vi "main.vi"() -> ()   [LabVIEW 2023, in "Vending_machine.lvlib"]
doc: "A vending machine"
uses:
  Vending_machine.lvlib
  Queue Opertaions.ctl
  Controls/Machine_data.ctl
  Controls/Cash.ctl
  Controls/Panel_states.ctl
  Controls/Read_Write.ctl
  <vilib>/Utility/error.llb/DialogType.ctl
  <vilib>/Utility/error.llb/Error Cluster From Error Code.vi
  <vilib>/ErrorRing/Error Ring.xnode
panel:
  in  "Gen_error":bool
  out "error out":errorcluster
  in  "error in (no error)":errorcluster
  in  "Reset Machine":bool
  out "Total cash":i32
  out "Total No. of cans":i32
  in  "Open Door":bool
  out "LED":bool
  in  "Cancel":bool
  in  "Sprite":bool
  in  "Fanta":bool
  in  "Coke":bool
  out "msg_box":string
  in  "5":bool
  in  "10":bool
  in  "20":bool
  in  "50":bool
  in  "100":bool
  # "Cash Selection"
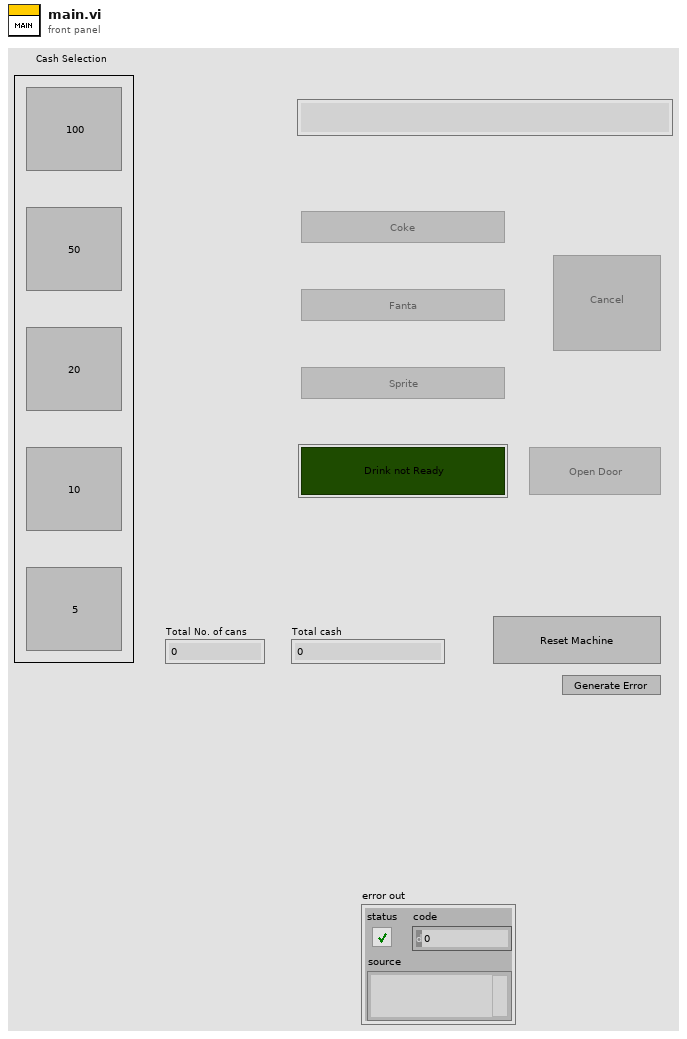
[diagram p1: front panel]
types:
  T1 = typedef "Vending_machine.lvlib/Queue Opertaions.ctl" = enum16{"Create", "Enqueue", "Enqueue N", "Flush", "Dequeue", "Destroy"}
  T2 = typedef "Vending_machine.lvlib/Machine_data.ctl" = cluster{"Cash":T3, "Panel_State":T4, "User_Cash":T3, "Drink":string, "Can_Count":i32, "Message_box":string, "LED":bool, "Last_Activity":timestamp, "Cash remaining":T3, "Drink_price":i32, "No_Activity_Limit(s)":dbl}
  T3 = typedef "Vending_machine.lvlib/Cash.ctl" = cluster{"100":i32, "50":i32, "20":i32, "10":i32, "5":i32}
  T4 = typedef "Vending_machine.lvlib/Panel_states.ctl" = cluster{"100":enum8{"Enabled", "Disabled", "Disabled and Grayed Out"}, "50":enum8{"Enabled", "Disabled", "Disabled and Grayed Out"}, "20":enum8{"Enabled", "Disabled", "Disabled and Grayed Out"}, "10":enum8{"Enabled", "Disabled", "Disabled and Grayed Out"}, "5":enum8{"Enabled", "Disabled", "Disabled and Grayed Out"}, "Cancel":enum8{"Enabled", "Disabled", "Disabled and Grayed Out"}, "Coke":enum8{"Enabled", "Disabled", "Disabled and Grayed Out"}, "Sprite":enum8{"Enabled", "Disabled", "Disabled and Grayed Out"}, "Fanta":enum8{"Enabled", "Disabled", "Disabled and Grayed Out"}, "Open_Door":enum8{"Enabled", "Disabled", "Disabled and Grayed Out"}}
  T5 = enum8{"Enabled", "Disabled", "Disabled and Grayed Out"}
  T6 = typedef "Vending_machine.lvlib/Read_Write.ctl" = enum16{"Read", "Write"}
  T7 = typedef "DialogType.ctl" = u16
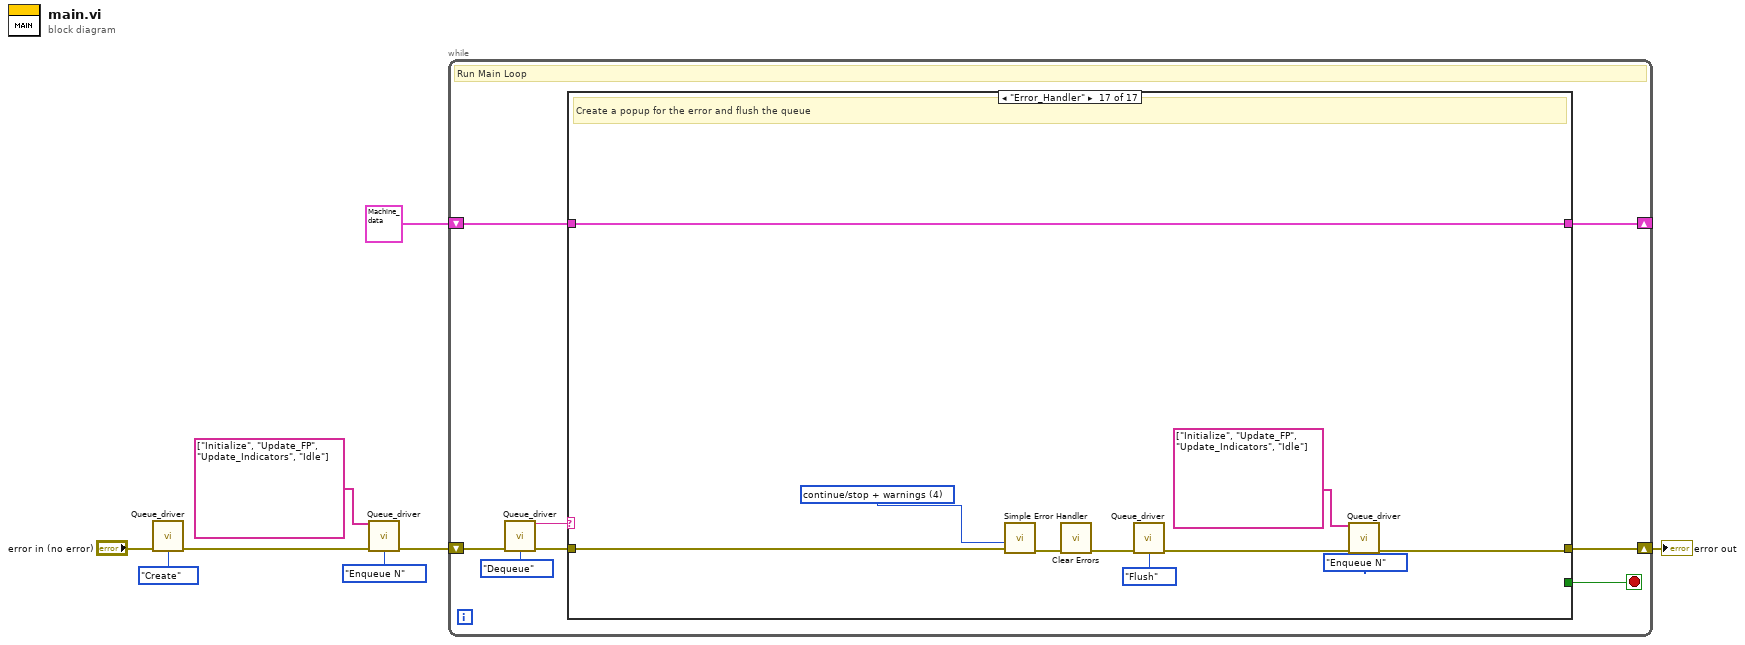
[diagram p0: block diagram]
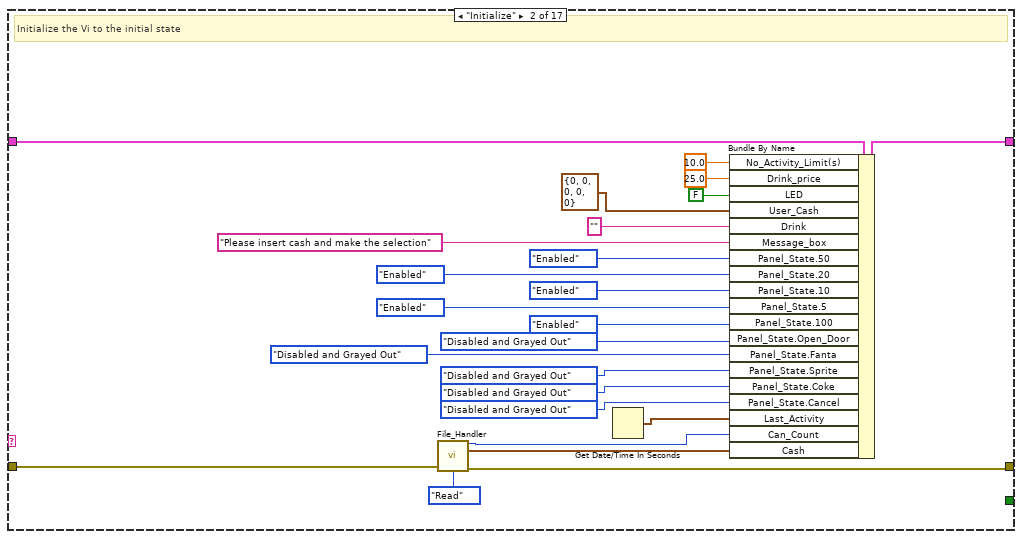
[diagram p3: hidden frame]
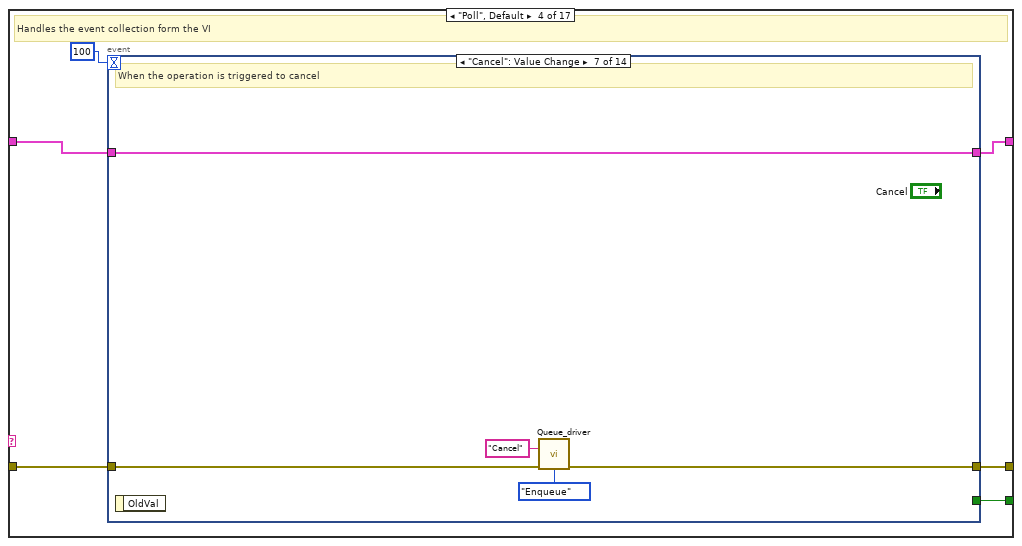
[diagram p5: hidden frame]
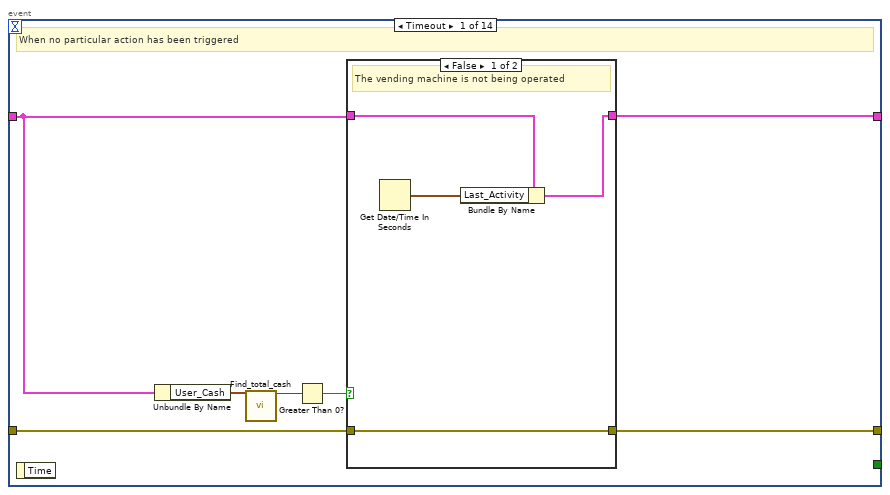
[diagram p6: hidden frame]
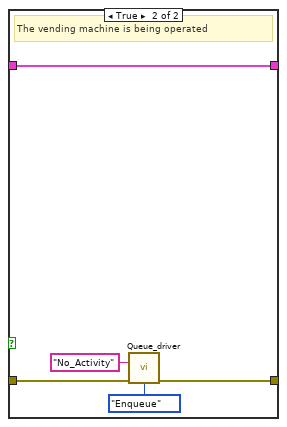
[diagram p7: hidden frame]
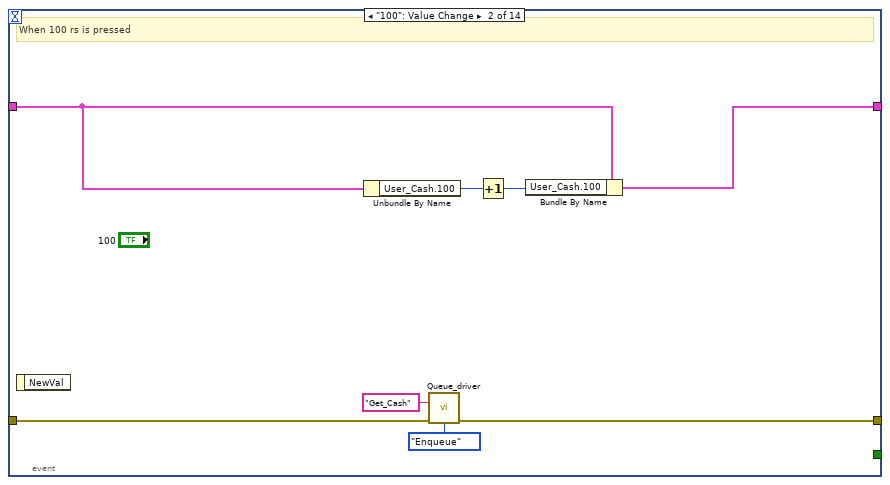
[diagram p8: hidden frame]
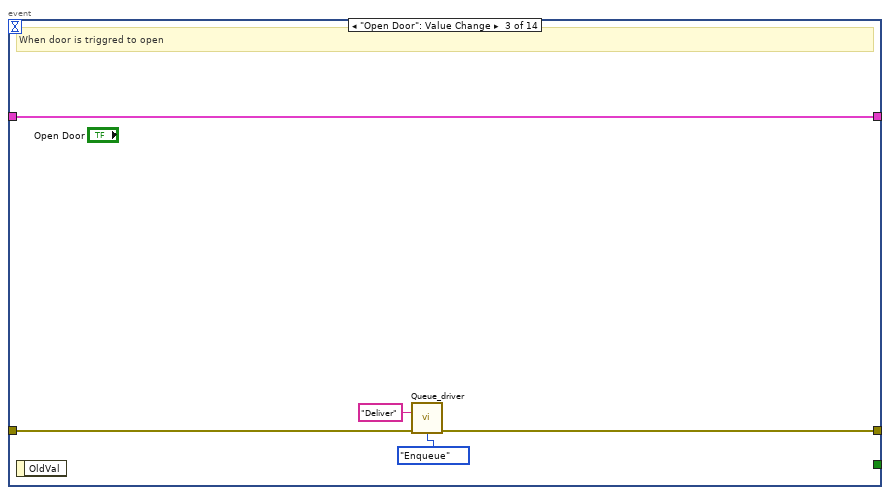
[diagram p9: hidden frame]
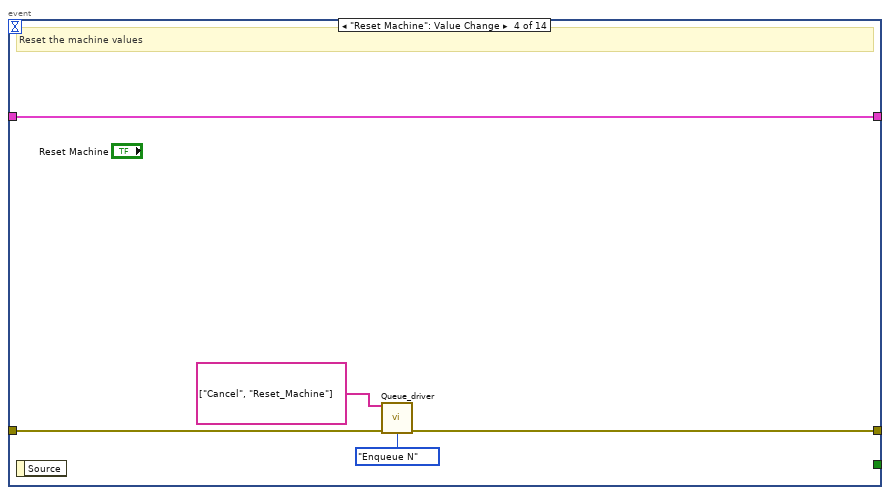
[diagram p10: hidden frame]
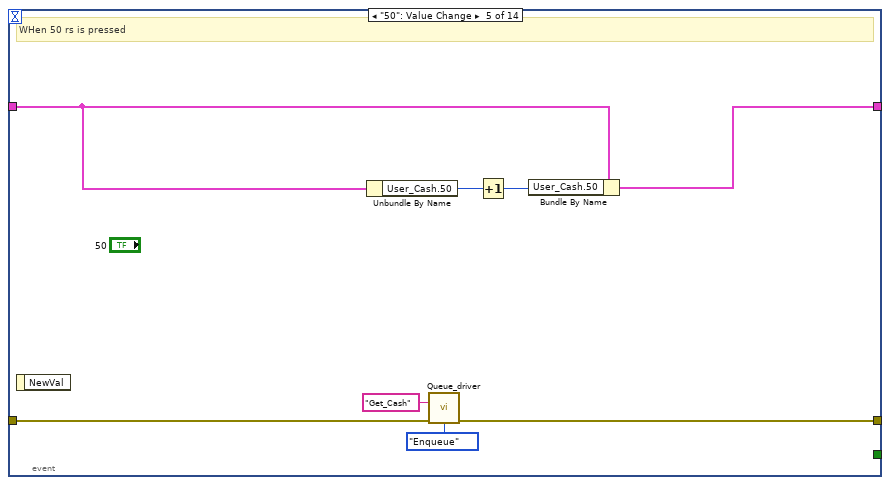
[diagram p11: hidden frame]
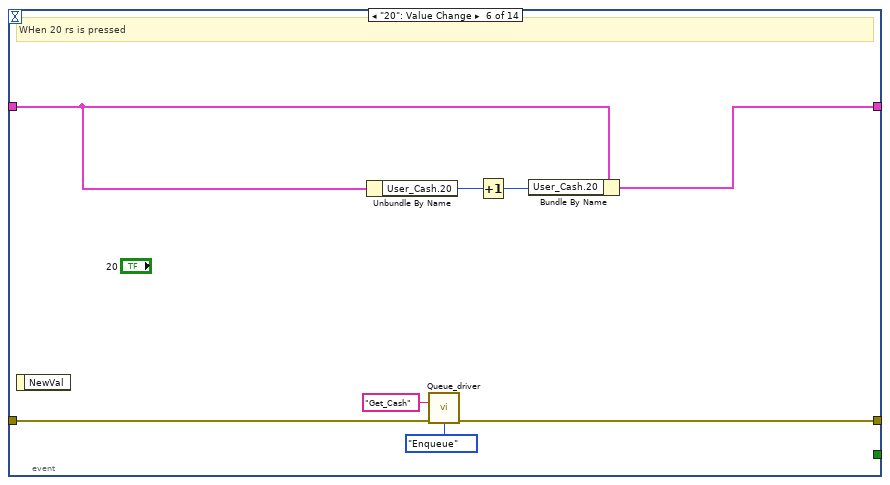
[diagram p12: hidden frame]
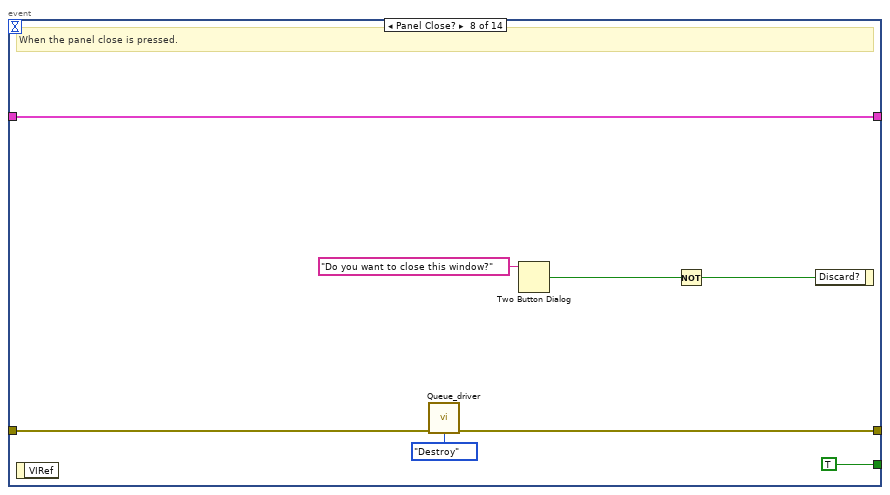
[diagram p13: hidden frame]
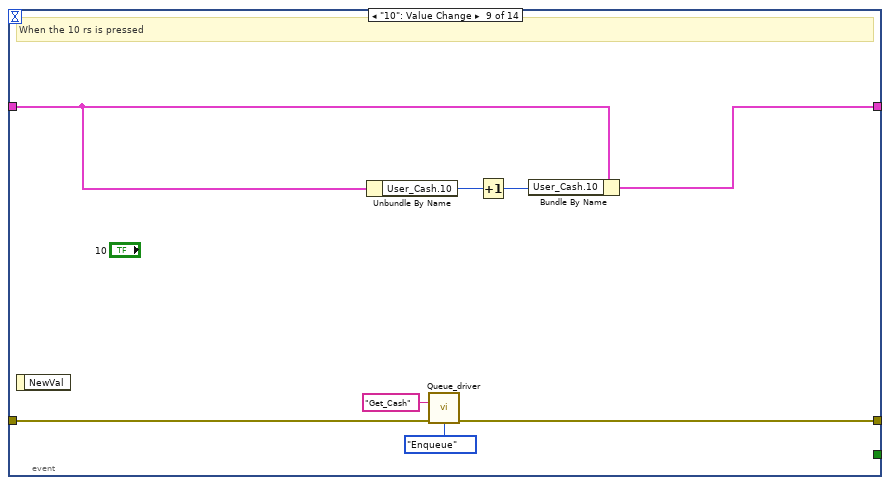
[diagram p14: hidden frame]
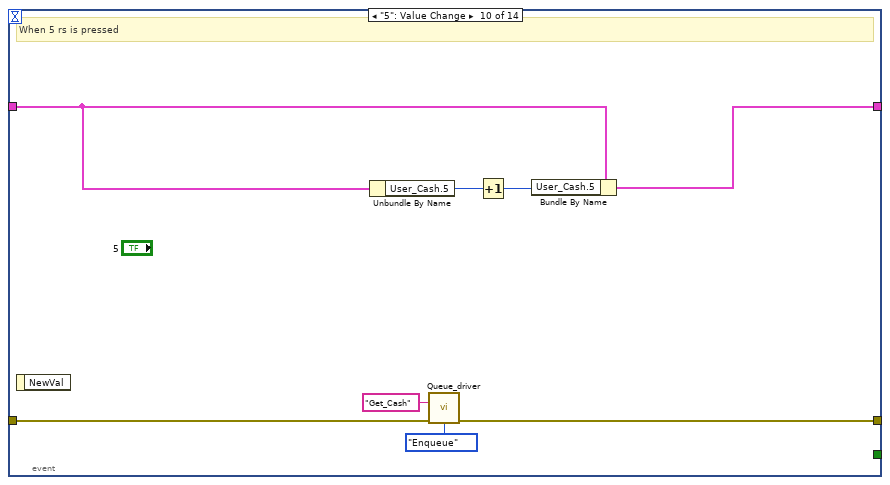
[diagram p15: hidden frame]
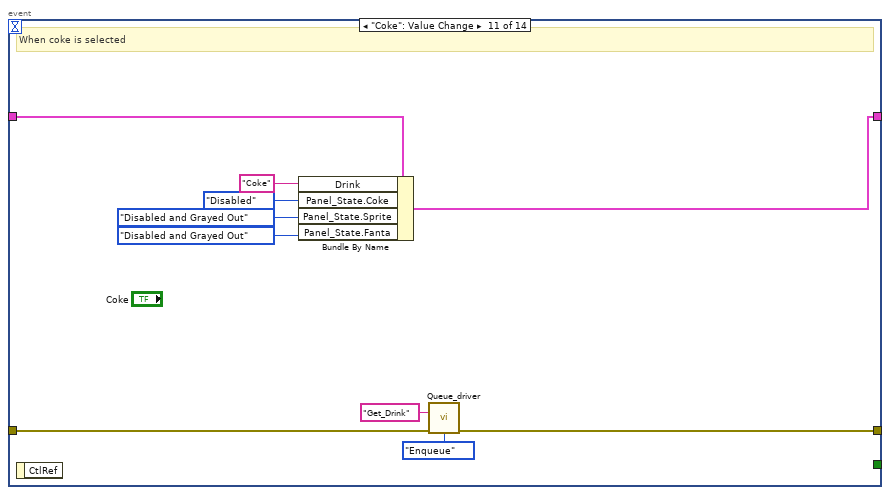
[diagram p16: hidden frame]
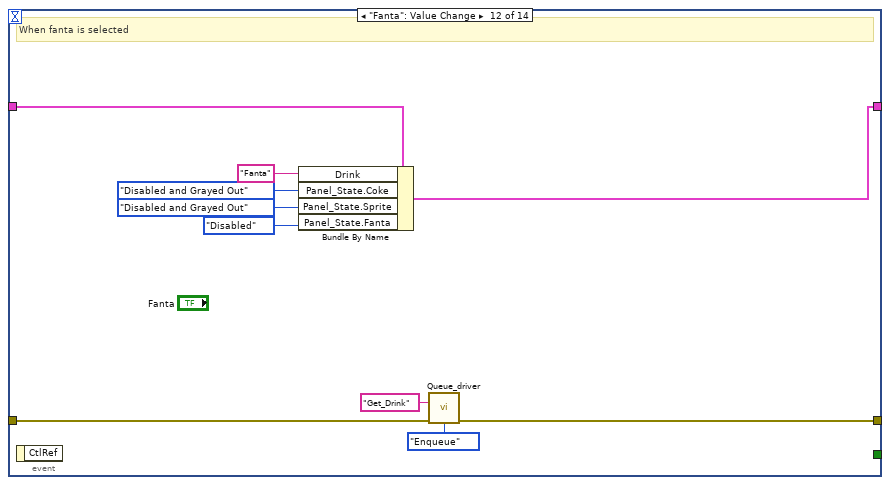
[diagram p17: hidden frame]
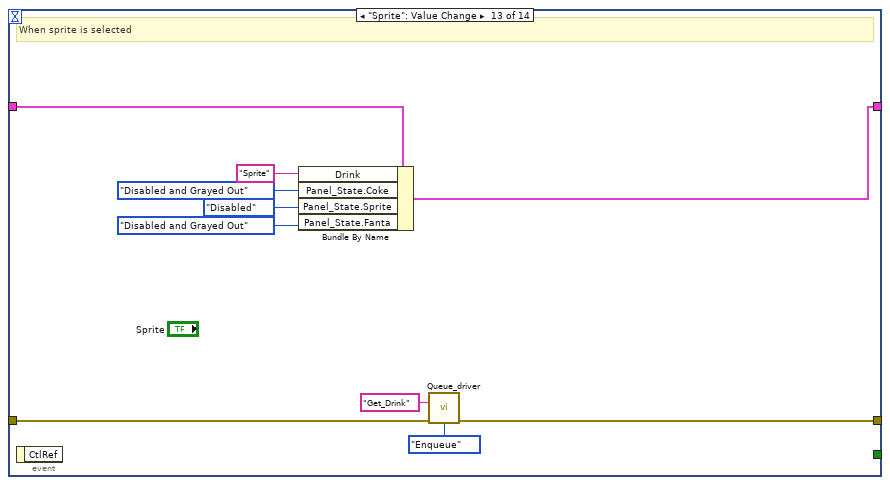
[diagram p18: hidden frame]
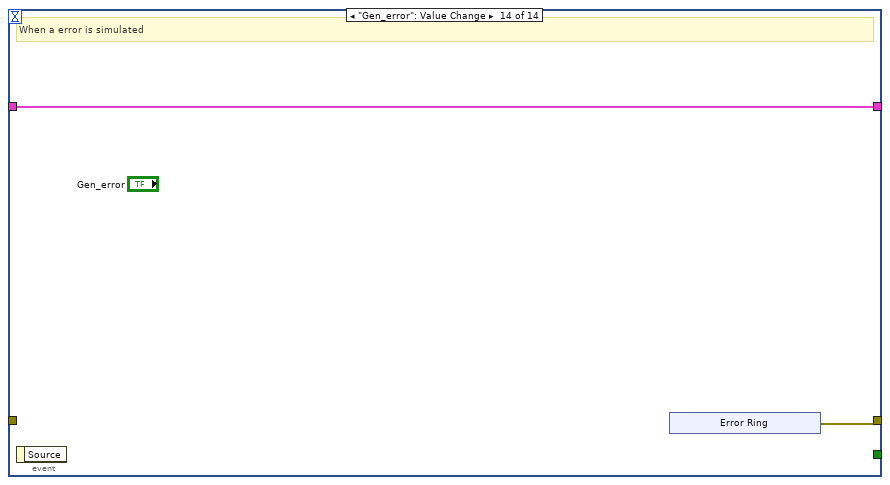
[diagram p19: hidden frame]
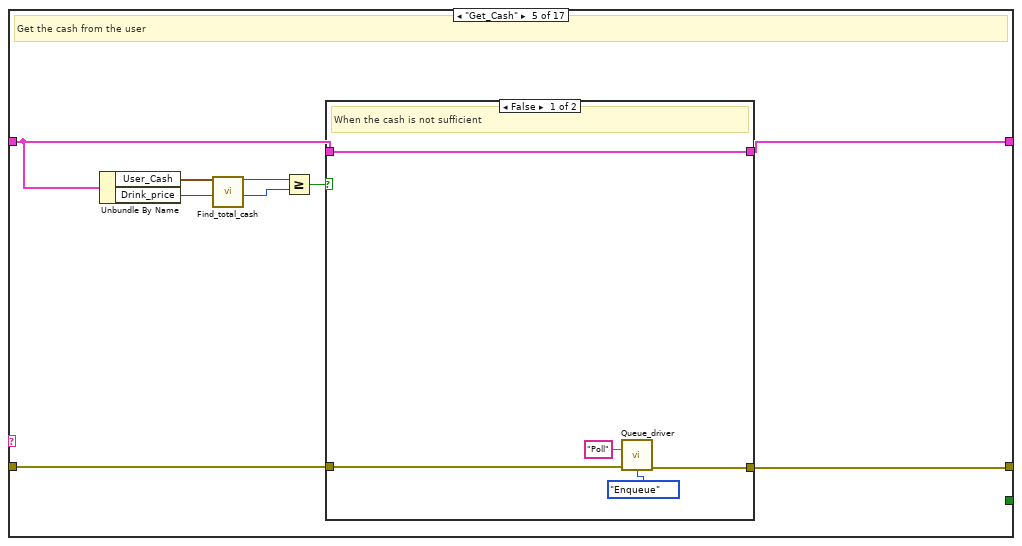
[diagram p20: hidden frame]
diagram:
  n1 = call "Queue_driver.vi"("error in (no error)"="error in (no error)", "Operations"=Queue_Opertaions."Create") -> ("error out"=w4:errorcluster)  [unwired: 12 in, 1 out]
  n2 = call "Queue_driver.vi"("Array Elements"=string[] ["Initialize", "Update_FP", "Update_Indicators", "Idle"], "error in (no error)"=w4, "Operations"=Queue_Opertaions."Enqueue N") -> ("error out"=w3:errorcluster)  [unwired: 11 in, 1 out]
  n3 = while {
    shift-right: [w13] -> _
    shift-left: T2 {"Cash"={"100"=0, "50"=0, "20"=0, "10"=0, "5"=0}, "Panel_State"={"100"=enum."Disabled and Grayed Out", "50"=enum."Disabled and Grayed Out", "20"=enum."Disabled and Grayed Out", "10"=enum."Disabled and Grayed Out", "5"=enum."Disabled and Grayed Out", "Cancel"=enum."Disabled and Grayed Out", "Coke"=enum."Disabled and Grayed Out", "Sprite"=enum."Disabled and Grayed Out", "Fanta"=enum."Disabled and Grayed Out", "Open_Door"=enum."Disabled and Grayed Out"}, "User_Cash"={"100"=0, "50"=0, "20"=0, "10"=0, "5"=0}, "Drink"="", "Can_Count"=0, "Message_box"="", "LED"=FALSE, "Last_Activity"=timestamp(0 s since 1904-01-01), "Cash remaining"={"100"=0, "50"=0, "20"=0, "10"=0, "5"=0}, "Drink_price"=0, "No_Activity_Limit(s)"=0.0} -> [w14]
    shift-right: [w15] -> w6
    shift-left: w3 -> [w16]
    stop <- w12 stop-if-true
    # "Run Main Loop"
    n4 = call "Queue_driver.vi"("error in (no error)"=w16, "Operations"=Queue_Opertaions."Dequeue") -> ("Element out"=w9:string, "error out"=w10:errorcluster)  [unwired: 12 in]
    n5 = case shown="\"Error_Handler\"" w9 {
      tunnel: w10 -> [w17 w41 w43 w49 w171 w205 w217 w229 w241 w261 w280 w298 w316 w323 w345 w350 w358]
      tunnel: [w17 w40 w43 w50 w170 w201 w216 w228 w240 w262 w281 w297 w316 w334 w345 w350 w354] -> w15
      tunnel: w14 -> [w18 w25 w44 w47 w169 w199 w220 w227 w239 w269 w283 w296 w317 w338 w349 w351 w361]
      tunnel: [w18 w42 w44 w46 w168 w198 w220 w227 w238 w269 w282 w295 w317 w338 w349 w351 w361] -> w13
      tunnel: [_ _ _ w45 _ _ _ _ _ _ _ _ _ _ _ _ _] -> w12
      frame "/***Init***/" {
        # "Contains cases related to intialising"
      }
      frame "Initialize" {
        # "Initialize the Vi to the initial state"
        n6 = call "File_Handler.vi"("error in (no error)"=w41, "Operations"=Read_Write."Read") -> ("Cans"=w37:i32, "Cash"=w38:T3, "error out"=w40:errorcluster)  [unwired: 11 in]
        n7 = Get Date/Time In Seconds() -> (seconds since 1Jan1904=w21:timestamp)
        n8 = Bundle By Name(cluster=w25, "No_Activity_Limit(s)"=10.0, "Drink_price"=25.0, "LED"=FALSE, "User_Cash"=T3 {"100"=0, "50"=0, "20"=0, "10"=0, "5"=0}, "Drink"="", "Message_box"="Please insert cash and make the selection", "Panel_State.50"=T5."Enabled", "Panel_State.20"=T5."Enabled", "Panel_State.10"=T5."Enabled", "Panel_State.5"=T5."Enabled", "Panel_State.100"=T5."Enabled", "Panel_State.Open_Door"=T5."Disabled and Grayed Out", "Panel_State.Fanta"=T5."Disabled and Grayed Out", "Panel_State.Sprite"=T5."Disabled and Grayed Out", "Panel_State.Coke"=T5."Disabled and Grayed Out", "Panel_State.Cancel"=T5."Disabled and Grayed Out", "Last_Activity"=w21, "Can_Count"=w37, "Cash"=w38) -> (w42:T2)
      }
      frame "/***Functionality***/" {
        # "Contains states related to functionlaity"
      }
      frame "Poll", Default {
        # "Handles the event collection form the VI"
        n9 = event shown="[6] \"Cancel\": Value Change" {
          selector: _ -> [_ _ _ _ _ _ _ _ _ _ _ _ _ _]
          dyn-events: _ -> [_ _ _ _ _ _ _ _ _ _ _ _ _ _]
          timeout: 100 -> [_ _ _ _ _ _ _ _ _ _ _ _ _ _]
          tunnel: [w56 w69 w76 w82 w87 w95 w102 w107 w116 w124 w132 w142 w152 w160] -> w50
          tunnel: w49 -> [w57 w70 w77 w83 w88 w96 w103 w113 w117 w125 w139 w149 w159 _]
          tunnel: w47 -> [w51 w74 w79 w84 w92 w100 w105 w111 w121 w129 w138 w148 w158 w161]
          tunnel: [w52 w73 w79 w84 w91 w99 w105 w111 w120 w128 w137 w147 w157 w161] -> w46
          tunnel: [_ _ _ _ _ _ _ TRUE _ _ _ _ _ _] -> w45
          event Timeout {
            # "When no particular action has been triggered"
            n10 = event-data() -> ()  [unwired: 1 in, 1 out]
            n11 = Unbundle By Name(w51) -> ("User_Cash"=w55:T3)
            n12 = call "Find_total_cash.vi"("Cash"=w55) -> ("Total_Cash"=w54:i32)  [unwired: 14 in]
            n13 = Greater Than 0?(x=w54) -> (x > 0?=w53:bool)
            n14 = case shown="False" w53 {
              tunnel: w57 -> [w61 w66]
              tunnel: [w61 w65] -> w56
              tunnel: [w58 w62] -> w52
              tunnel: w51 -> [w59 w62]
              frame False {
                # "The vending machine is not being operated"
                n15 = Get Date/Time In Seconds() -> (seconds since 1Jan1904=w60:timestamp)
                n16 = Bundle By Name(cluster=w59, "Last_Activity"=w60) -> (w58:T2)
              }
              frame True {
                # "The vending machine is being operated"
                n17 = call "Queue_driver.vi"("Element in"="No_Activity", "error in (no error)"=w66, "Operations"=Queue_Opertaions."Enqueue") -> ("error out"=w65:errorcluster)  [unwired: 11 in, 1 out]
              }
            }
          }
          event "100": Value Change {
            # "When 100 rs is pressed"
            n18 = event-data() -> ()  [unwired: 1 in, 1 out]
            n19 = Unbundle By Name(w74) -> ("User_Cash.100"=w72:i32)
            n20 = call "Queue_driver.vi"("Element in"="Get_Cash", "error in (no error)"=w70, "Operations"=Queue_Opertaions."Enqueue") -> ("error out"=w69:errorcluster)  [unwired: 11 in, 1 out]
            n21 = Increment(x=w72) -> (x+1=w71:i32)
            n22 = Bundle By Name(cluster=w74, "User_Cash.100"=w71) -> (w73:T2)
          }
          event "Open Door": Value Change {
            # "When door is triggred to open"
            n23 = event-data() -> ()  [unwired: 1 in, 1 out]
            n24 = call "Queue_driver.vi"("Element in"="Deliver", "error in (no error)"=w77, "Operations"=Queue_Opertaions."Enqueue") -> ("error out"=w76:errorcluster)  [unwired: 11 in, 1 out]
          }
          event "Reset Machine": Value Change {
            # "Reset the machine values"
            n25 = event-data() -> ()  [unwired: 1 in, 1 out]
            n26 = call "Queue_driver.vi"("Array Elements"=string[] ["Cancel", "Reset_Machine"], "error in (no error)"=w83, "Operations"=Queue_Opertaions."Enqueue N") -> ("error out"=w82:errorcluster)  [unwired: 11 in, 1 out]
          }
          event "50": Value Change {
            # "WHen 50 rs is pressed"
            n27 = event-data() -> ()  [unwired: 1 in, 1 out]
            n28 = Unbundle By Name(w92) -> ("User_Cash.50"=w90:i32)
            n29 = call "Queue_driver.vi"("Element in"="Get_Cash", "error in (no error)"=w88, "Operations"=Queue_Opertaions."Enqueue") -> ("error out"=w87:errorcluster)  [unwired: 11 in, 1 out]
            n30 = Increment(x=w90) -> (x+1=w89:i32)
            n31 = Bundle By Name(cluster=w92, "User_Cash.50"=w89) -> (w91:T2)
          }
          event "20": Value Change {
            # "WHen 20 rs is pressed"
            n32 = event-data() -> ()  [unwired: 1 in, 1 out]
            n33 = Unbundle By Name(w100) -> ("User_Cash.20"=w98:i32)
            n34 = call "Queue_driver.vi"("Element in"="Get_Cash", "error in (no error)"=w96, "Operations"=Queue_Opertaions."Enqueue") -> ("error out"=w95:errorcluster)  [unwired: 11 in, 1 out]
            n35 = Increment(x=w98) -> (x+1=w97:i32)
            n36 = Bundle By Name(cluster=w100, "User_Cash.20"=w97) -> (w99:T2)
          }
          event "Cancel": Value Change {
            # "When the operation is triggered to cancel"
            n37 = event-data() -> ()  [unwired: 1 in, 1 out]
            n38 = call "Queue_driver.vi"("Element in"="Cancel", "error in (no error)"=w103, "Operations"=Queue_Opertaions."Enqueue") -> ("error out"=w102:errorcluster)  [unwired: 11 in, 1 out]
          }
          event Panel Close? {
            # "When the panel close is pressed."
            n39 = event-data() -> ()  [unwired: 1 in, 1 out]
            n40 = call "Queue_driver.vi"("error in (no error)"=w113, "Operations"=Queue_Opertaions."Destroy") -> ("error out"=w107:errorcluster)  [unwired: 12 in, 1 out]
            n41 = Two Button Dialog(message="Do you want to close this window?") -> (T button?=w109:bool)  [unwired: 2 in]
            n42 = Not(x=w109) -> (.not. x?=w108:bool)
            n43 = event-data("Discard?"=w108) -> ()  [unwired: 1 in, 1 out]
          }
          event "10": Value Change {
            # "When the 10 rs is pressed"
            n44 = event-data() -> ()  [unwired: 1 in, 1 out]
            n45 = Unbundle By Name(w121) -> ("User_Cash.10"=w119:i32)
            n46 = call "Queue_driver.vi"("Element in"="Get_Cash", "error in (no error)"=w117, "Operations"=Queue_Opertaions."Enqueue") -> ("error out"=w116:errorcluster)  [unwired: 11 in, 1 out]
            n47 = Increment(x=w119) -> (x+1=w118:i32)
            n48 = Bundle By Name(cluster=w121, "User_Cash.10"=w118) -> (w120:T2)
          }
          event "5": Value Change {
            # "When 5 rs is pressed"
            n49 = event-data() -> ()  [unwired: 1 in, 1 out]
            n50 = Unbundle By Name(w129) -> ("User_Cash.5"=w127:i32)
            n51 = call "Queue_driver.vi"("Element in"="Get_Cash", "error in (no error)"=w125, "Operations"=Queue_Opertaions."Enqueue") -> ("error out"=w124:errorcluster)  [unwired: 11 in, 1 out]
            n52 = Increment(x=w127) -> (x+1=w126:i32)
            n53 = Bundle By Name(cluster=w129, "User_Cash.5"=w126) -> (w128:T2)
          }
          event "Coke": Value Change {
            # "When coke is selected"
            n54 = event-data() -> ()  [unwired: 1 in, 1 out]
            n55 = Bundle By Name(cluster=w138, "Drink"="Coke", "Panel_State.Coke"=T5."Disabled", "Panel_State.Sprite"=T5."Disabled and Grayed Out", "Panel_State.Fanta"=T5."Disabled and Grayed Out") -> (w137:T2)
            n56 = call "Queue_driver.vi"("Element in"="Get_Drink", "error in (no error)"=w139, "Operations"=Queue_Opertaions."Enqueue") -> ("error out"=w132:errorcluster)  [unwired: 11 in, 1 out]
          }
          event "Fanta": Value Change {
            # "When fanta is selected"
            n57 = event-data() -> ()  [unwired: 1 in, 1 out]
            n58 = Bundle By Name(cluster=w148, "Drink"="Fanta", "Panel_State.Coke"=T5."Disabled and Grayed Out", "Panel_State.Sprite"=T5."Disabled and Grayed Out", "Panel_State.Fanta"=T5."Disabled") -> (w147:T2)
            n59 = call "Queue_driver.vi"("Element in"="Get_Drink", "error in (no error)"=w149, "Operations"=Queue_Opertaions."Enqueue") -> ("error out"=w142:errorcluster)  [unwired: 11 in, 1 out]
          }
          event "Sprite": Value Change {
            # "When sprite is selected"
            n60 = event-data() -> ()  [unwired: 1 in, 1 out]
            n61 = Bundle By Name(cluster=w158, "Drink"="Sprite", "Panel_State.Coke"=T5."Disabled and Grayed Out", "Panel_State.Sprite"=T5."Disabled", "Panel_State.Fanta"=T5."Disabled and Grayed Out") -> (w157:T2)
            n62 = call "Queue_driver.vi"("Element in"="Get_Drink", "error in (no error)"=w159, "Operations"=Queue_Opertaions."Enqueue") -> ("error out"=w152:errorcluster)  [unwired: 11 in, 1 out]
          }
          event "Gen_error": Value Change {
            # "When a error is simulated"
            n63 = event-data() -> ()  [unwired: 1 in, 1 out]
            n64 = xnode "Error Ring"() -> ("error out"=w160:errorcluster)
          }
        }
      }
      frame "Get_Cash" {
        # "Get the cash from the user"
        n65 = Unbundle By Name(w169) -> ("User_Cash"=w174:T3, "Drink_price"=w167:i32)
        n66 = call "Find_total_cash.vi"("Cash"=w174) -> ("Total_Cash"=w173:i32)  [unwired: 14 in]
        n67 = Greater Or Equal?(x=w173, y=w167) -> (x >= y?=w172:bool)
        n68 = case shown="False" w172 {
          tunnel: w171 -> [w178 w195]
          tunnel: [w177 w194] -> w170
          tunnel: w169 -> [w179 w193]
          tunnel: [w179 w192] -> w168
          frame False {
            # "When the cash is not sufficient"
            n69 = call "Queue_driver.vi"("Element in"="Poll", "error in (no error)"=w178, "Operations"=Queue_Opertaions."Enqueue") -> ("error out"=w177:errorcluster)  [unwired: 11 in, 1 out]
          }
          frame True {
            # "When the user has given more than minimum amount"
            n70 = call "Queue_driver.vi"("Array Elements"=string[] ["Update_FP", "Update_Indicators", "Check_Change", "Check_Drink", "Get_Drink"], "error in (no error)"=w195, "Operations"=Queue_Opertaions."Enqueue N") -> ("error out"=w194:errorcluster)  [unwired: 11 in, 1 out]
            n71 = Bundle By Name(cluster=w193, "Panel_State.100"=T5."Disabled and Grayed Out", "Panel_State.50"=T5."Disabled and Grayed Out", "Panel_State.20"=T5."Disabled and Grayed Out", "Panel_State.10"=T5."Disabled and Grayed Out", "Panel_State.5"=T5."Disabled and Grayed Out", "Panel_State.Cancel"=T5."Enabled", "Panel_State.Coke"=T5."Enabled", "Panel_State.Sprite"=T5."Enabled", "Panel_State.Fanta"=T5."Enabled", "Message_box"="Cash inserted!!, Select the drink") -> (w192:T2)
          }
        }
      }
      frame "Check_Change" {
        # "Check whether there is change is machine"
        n72 = Unbundle By Name(w199) -> ("User_Cash"=w203:T3, "Cash"=w204:T3, "Drink_price"=w196:i32)
        n73 = call "calculate_change.vi"("User_cash"=w203, "Machine_cash"=w204, "Amount"=w196, "error in (no error)"=w205) -> ("Machine_cash"=w197:T3, "Has_change"=w200:bool, "error in (no error) 2"=w202:errorcluster)  [unwired: 8 in, 1 out]
        n74 = case shown="False" w200 {
          tunnel: w202 -> [w209 w215]
          tunnel: [w211 w215] -> w201
          tunnel: w199 -> [w206 w214]
          tunnel: [w206 w213] -> w198
          tunnel: w197 -> [_ w212]
          frame False {
            # "No change is present"
            n75 = One Button Dialog(message="We apologise for inconvinence, But no change is present at this moment, \nKindly collect your cash") -> ()  [unwired: 1 in, 1 out]
            n76 = call "Queue_driver.vi"("Array Elements"=string[] ["Initialize", "Update_FP", "Update_Indicators", "Get_Cash"], "error in (no error)"=w209, "Operations"=Queue_Opertaions."Enqueue N") -> ("error out"=w211:errorcluster)  [unwired: 11 in, 1 out]
          }
          frame True {
            # "Change is present"
            n77 = Bundle By Name(cluster=w214, "Cash remaining"=w212) -> (w213:T2)
          }
        }
      }
      frame "Check_Drink" {
        # "Check whether drink is present in machine"
        n78 = Unbundle By Name(w220) -> ("Can_Count"=w219:i32)
        n79 = Greater Than 0?(x=w219) -> (x > 0?=w218:bool)
        n80 = case shown="True" w218 {
          tunnel: w217 -> [w222 w226]
          tunnel: [w221 w226] -> w216
          frame False {
            # "Drink is present"
            n81 = call "Queue_driver.vi"("Array Elements"=string[] ["Initialize", "Update_FP", "Update_Indicators", "Get_Cash"], "error in (no error)"=w222, "Operations"=Queue_Opertaions."Enqueue N") -> ("error out"=w221:errorcluster)  [unwired: 11 in, 1 out]
            n82 = One Button Dialog(message="We apologise for inconvinence, But No drink is present at this moment, \nKindly collect your cash") -> ()  [unwired: 1 in, 1 out]
          }
          frame True {
            # "Drink is absent"
          }
        }
      }
      frame "Cancel" {
        # "When the operation is to be cancelled"
        n83 = Unbundle By Name(w227) -> ("User_Cash"=w234:T3)
        n84 = call "Find_total_cash.vi"("Cash"=w234) -> ("Total_Cash"=w236:i32)  [unwired: 14 in]
        n85 = Format Into String(format string="\\nKindly Collect Your %d Ruppees", initial string="The operations has be cancelled successfully" ("message"), error in=w229, w236) -> (resulting string=w232:string, error out=w235:errorcluster)
        n86 = One Button Dialog(message=w232) -> ()  [unwired: 1 in, 1 out]
        n87 = call "Queue_driver.vi"("Array Elements"=string[] ["Initialize", "Update_FP", "Update_Indicators", "Get_Cash"], "error in (no error)"=w235, "Operations"=Queue_Opertaions."Enqueue N") -> ("error out"=w228:errorcluster)  [unwired: 11 in, 1 out]
      }
      frame "Get_Drink" {
        # "Get the selected drink"
        n88 = Unbundle By Name(w239) -> ("Drink"=w243:string)
        n89 = Empty String/Path?(string/path=w243) -> (empty?=w242:bool)
        n90 = case shown="True" w242 {
          tunnel: w241 -> [w250 w258]
          tunnel: [w249 w257] -> w240
          tunnel: w239 -> [w253 w255]
          tunnel: [w252 w255] -> w238
          frame False {
            # "When a drink is selected"
            n91 = Get Date/Time In Seconds() -> (seconds since 1Jan1904=w244:timestamp)
            n92 = Bundle By Name(cluster=w253, "Panel_State.Cancel"=T5."Disabled and Grayed Out", "LED"=TRUE ("Panel_State.LED"), "Panel_State.Open_Door"=T5."Enabled", "Last_Activity"=w244) -> (w252:T2)
            n93 = call "Queue_driver.vi"("Array Elements"=string[] ["Update_FP", "Update_Indicators"], "error in (no error)"=w250, "Operations"=Queue_Opertaions."Enqueue N") -> ("error out"=w249:errorcluster)  [unwired: 11 in, 1 out]
          }
          frame True {
            # "When a drink is not selected"
            n94 = call "Queue_driver.vi"("Array Elements"=string[] ["Poll"], "error in (no error)"=w258, "Operations"=Queue_Opertaions."Enqueue N") -> ("error out"=w257:errorcluster)  [unwired: 11 in, 1 out]
          }
        }
      }
      frame "Reset_Machine" {
        # "When the machine is to be reset"
        n95 = call "Queue_driver.vi"("error in (no error)"=w261, "Operations"=Queue_Opertaions."Flush") -> ("error out"=w260:errorcluster)  [unwired: 12 in, 1 out]
        n96 = call "Queue_driver.vi"("Array Elements"=string[] ["Initialize", "Update_FP", "Update_Indicators", "Get_Cash"], "error in (no error)"=w260, "Operations"=Queue_Opertaions."Enqueue N") -> ("error out"=w265:errorcluster)  [unwired: 11 in, 1 out]
        n97 = call "File_Handler.vi"("Cans"=100, "Cash"=T3 {"100"=0, "50"=0, "20"=0, "10"=0, "5"=200}, "error in (no error)"=w265, "Operations"=Read_Write."Write") -> ("error out"=w262:errorcluster)  [unwired: 9 in, 2 out]
      }
      frame "Deliver" {
        # "When the selected drink is be deliverd vi Door"
        n98 = Unbundle By Name(w283) -> ("Can_Count"=w288:i32, "Cash remaining"=w285:T3, "User_Cash"=w276:T3)
        n99 = call "Queue_driver.vi"("Array Elements"=string[] ["Initialize", "Update_FP", "Update_Indicators", "Get_Cash"], "error in (no error)"=w280, "Operations"=Queue_Opertaions."Enqueue N") -> ("error out"=w284:errorcluster)  [unwired: 11 in, 1 out]
        n100 = call "Find_total_cash.vi"("Cash"=w276) -> ("Total_Cash"=w275:i32)  [unwired: 14 in]
        n101 = Decrement(x=w288) -> (x-1=w286:i32)
        n102 = Subtract(x=w275, y=25) -> (x-y=w271:i32)
        n103 = Number To Decimal String(number=w271, width (-)=i16 0) -> (decimal integer string=w274:string)
        n104 = Concatenate Strings("Kindly collect your drink and change Rs. " ("message"), w274) -> (w272:string)
        n105 = One Button Dialog(message=w272) -> ()  [unwired: 1 in, 1 out]
        n106 = call "File_Handler.vi"("Cans"=w286, "Cash"=w285, "error in (no error)"=w284, "Operations"=Read_Write."Write") -> ("error out"=w281:errorcluster)  [unwired: 9 in, 2 out]
        n107 = Bundle By Name(cluster=w283, "Can_Count"=w286, "Cash"=w285) -> (w282:T2)
      }
      frame "No_Activity" {
        # "When there is no activity for a certain time"
        n108 = Unbundle By Name(w296) -> ("Last_Activity"=w291:timestamp, "No_Activity_Limit(s)"=w289:dbl, "User_Cash"=w290:T3)
        n109 = Get Date/Time In Seconds() -> (seconds since 1Jan1904=w292:timestamp)
        n110 = Subtract(x=w292, y=w291) -> (x-y=w294:dbl)
        n111 = Greater Or Equal?(x=w294, y=w289) -> (x >= y?=w293:bool)
        n112 = case shown="False" w293 {
          tunnel: [w300 w306] -> w297
          tunnel: w298 -> [w300 w307]
          tunnel: w290 -> [_ w308]
          tunnel: w296 -> [w299 w305]
          tunnel: [w299 w302] -> w295
          frame False {
            # "WHen the limit has not been exceeded"
          }
          frame True {
            # "When the limit has been exceeded"
            n113 = call "Find_total_cash.vi"("Cash"=w308) -> ("Total_Cash"=w313:i32)  [unwired: 14 in]
            n114 = Format Into String(format string="\\nKindly Collect Your %d Ruppees", initial string="No user activity detected. Cancelling the operation." ("message"), error in=w307, w313) -> (resulting string=w315:string, error out=w314:errorcluster)
            n115 = Get Date/Time In Seconds() -> (seconds since 1Jan1904=w301:timestamp)
            n116 = One Button Dialog(message=w315) -> ()  [unwired: 1 in, 1 out]
            n117 = Bundle By Name(cluster=w305, "Last_Activity"=w301) -> (w302:T2)
            n118 = call "Queue_driver.vi"("error in (no error)"=w314, "Operations"=Queue_Opertaions."Flush") -> ("error out"=w304:errorcluster)  [unwired: 12 in, 1 out]
            n119 = call "Queue_driver.vi"("Array Elements"=string[] ["Initialize", "Update_FP", "Update_Indicators", "Get_Cash"], "error in (no error)"=w304, "Operations"=Queue_Opertaions."Enqueue N") -> ("error out"=w306:errorcluster)  [unwired: 11 in, 1 out]
          }
        }
      }
      frame "/***FP operations***/" {
        # "Operation related to front panel"
      }
      frame "Update_FP" {
        # "Update the front panel elements"
        n120 = Unbundle By Name(w338) -> ("Panel_State.5"=w333:T5, "Panel_State.10"=w332:T5, "Panel_State.20"=w331:T5, "Panel_State.50"=w330:T5, "Panel_State.100"=w329:T5, "Panel_State.Cancel"=w328:T5, "Panel_State.Coke"=w327:T5, "Panel_State.Sprite"=w326:T5, "Panel_State.Fanta"=w325:T5, "Panel_State.Open_Door"=w324:T5)
        n121 = property on="Open Door" class="Bool"(error in=w323, "DisabledEnum"=w324) -> (error out=w322:errorcluster)  [unwired: 1 in, 1 out]
        n122 = property on="Fanta" class="Bool"(error in=w322, "DisabledEnum"=w325) -> (error out=w321:errorcluster)  [unwired: 1 in, 1 out]
        n123 = property on="Sprite" class="Bool"(error in=w321, "DisabledEnum"=w326) -> (error out=w320:errorcluster)  [unwired: 1 in, 1 out]
        n124 = property on="Coke" class="Bool"(error in=w320, "DisabledEnum"=w327) -> (error out=w319:errorcluster)  [unwired: 1 in, 1 out]
        n125 = property on="Cancel" class="Bool"(error in=w319, "DisabledEnum"=w328) -> (error out=w318:errorcluster)  [unwired: 1 in, 1 out]
        n126 = property on="100" class="Bool"(error in=w318, "DisabledEnum"=w329) -> (error out=w339:errorcluster)  [unwired: 1 in, 1 out]
        n127 = property on="50" class="Bool"(error in=w339, "DisabledEnum"=w330) -> (error out=w337:errorcluster)  [unwired: 1 in, 1 out]
        n128 = property on="20" class="Bool"(error in=w337, "DisabledEnum"=w331) -> (error out=w336:errorcluster)  [unwired: 1 in, 1 out]
        n129 = property on="10" class="Bool"(error in=w336, "DisabledEnum"=w332) -> (error out=w335:errorcluster)  [unwired: 1 in, 1 out]
        n130 = property on="5" class="Bool"(error in=w335, "DisabledEnum"=w333) -> (error out=w334:errorcluster)  [unwired: 1 in, 1 out]
      }
      frame "Update_Indicators" {
        # "Update the indicators in front panel"
        n131 = Unbundle By Name(w349) -> ("Message_box"=→"msg_box":string, "Can_Count"=→"Total No. of cans":i32, "Cash"=w346:T3, "User_Cash"=w343:T3, "LED"=→"LED":bool)
        n132 = call "Find_total_cash.vi"("Cash"=w346) -> ("Total_Cash"=w341:i32)  [unwired: 14 in]
        n133 = call "Find_total_cash.vi"("Cash"=w343) -> ("Total_Cash"=w342:i32)  [unwired: 14 in]
        n134 = Add(x=w341, y=w342) -> (x+y=→"Total cash":i32)
      }
      frame "/***Error_Handling***/" {
        # "Error handling states"
      }
      frame "Error_Handler" {
        w359 = T7 4 items=["no dialog", "OK message", "continue or stop message", "OK message + warnings", "continue/stop + warnings"] ("type of dialog (OK msg:1)")
        # "Create a popup for the error and flush the queue"
        n135 = call <vilib>:"Simple Error Handler.vi"("type of dialog (OK msg:1)"=w359, "error in (no error)"=w358) -> ("error out"=w360:errorcluster)  [unwired: 3 in, 4 out]
        n136 = call <vilib>:"Clear Errors.vi"("error in (no error)"=w360) -> ("error out"=w357:errorcluster)  [unwired: 5 in, 1 out]
        n137 = call "Queue_driver.vi"("error in (no error)"=w357, "Operations"=Queue_Opertaions."Flush") -> ("error out"=w356:errorcluster)  [unwired: 12 in, 1 out]
        n138 = call "Queue_driver.vi"("Array Elements"=string[] ["Initialize", "Update_FP", "Update_Indicators", "Idle"], "error in (no error)"=w356, "Operations"=Queue_Opertaions."Enqueue N") -> ("error out"=w354:errorcluster)  [unwired: 11 in, 1 out]
      }
    }
  }
  "error out" <- w6
